vi "VI1.vi"() -> ()   [LabVIEW 2012]
uses:
  <vilib>/rvi/eio/common/nirviEmuTemplateMethod_errors.vi
  <vilib>/eio/EIONode/EIONode.xnode
panel:
  out "Mod2/AI0":i16
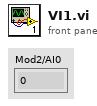
[diagram p1: front panel]
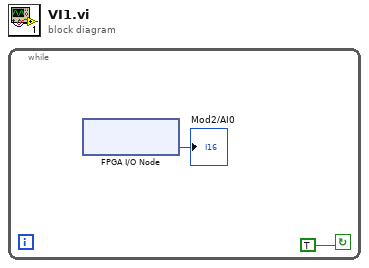
[diagram p0: block diagram]
diagram:
  n1 = while {
    stop <- TRUE continue-if-true
    n2 = xnode "FPGA I/O Node"() -> ("Mod2/AI0"=→"Mod2/AI0":i16)  [unwired: 1 in, 1 out]
  }
